vi "Cleanup.vi"(8 "error in (no error)":errorcluster, 11 "Manager in":refnum<class "Manager.lvclass">) -> (0 "error out":errorcluster)   [LabVIEW 2020, in "Stream-Simple-Msg.lvlib" / "Manager.lvclass"]
doc: "Closes all connected endpoints and cleans up all resources used by the specified messaging manager."
uses:
  Manager.lvclass
  Manager.lvclass/Manager.ctl
  <vilib>/IlluminatedG/lv-stream/Endpoint/Endpoint.lvclass
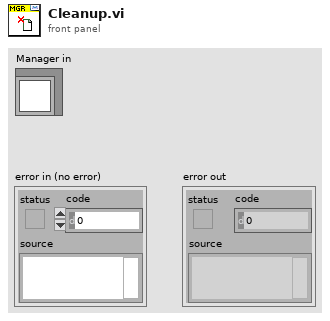
[diagram p1: front panel]
types:
  T1 = typedef "Stream-Simple-Msg.lvlib/Manager.lvclass/Ref Data.ctl" = cluster{"Message Callbacks":map{string, T2[]}, "Endpoints":map{string, refnum<class "Endpoint.lvclass">}, "Stream Endpoints":refnum<class "Endpoint.lvclass">[], "State Callbacks":T3[]}
  T2 = typedef "Stream-Simple-Msg.lvlib/Manager.lvclass/Callback.ctl" = cluster{"VI":refnum<vi>, "Owner":refnum<class>}
  T3 = typedef "Stream-Simple-Msg.lvlib/Manager.lvclass/State Callback.ctl" = cluster{"Owner":refnum<class>, "VI":refnum<vi>}
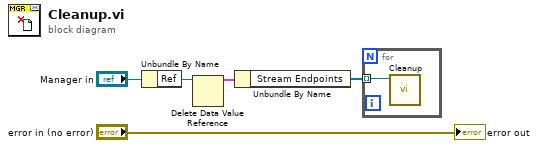
[diagram p0: block diagram]
diagram:
  n1 = Unbundle By Name("Manager in") -> ("Ref"=w3:refnum<data-value>)
  n2 = Delete Data Value Reference(data value reference=w3) -> (data value=w2:T1)  [unwired: 1 in, 1 out]
  n3 = Unbundle By Name(w2) -> ("Stream Endpoints"=w1:refnum<class "Endpoint.lvclass">[])
  n4 = for {
    tunnel: w1 -> [w6] mode=indexing
    n5 = call-dynamic "Cleanup.vi"("Endpoint in"=w6) -> ()  [unwired: 10 in, 1 out]
  }
  "error out" <- "error in (no error)"
